vi "Load Shared Library.vi"(7 "Unload":bool, 8 "Error In":errorcluster, 11 "LabPack Shared Library In":path=path "") -> (0 "Error Out":errorcluster, 2 "Version":string, 3 "LabPack Shared Library Out":path)   [LabVIEW 2017, in "LabPack.lvlib"]
uses:
  LabPack.lvlib
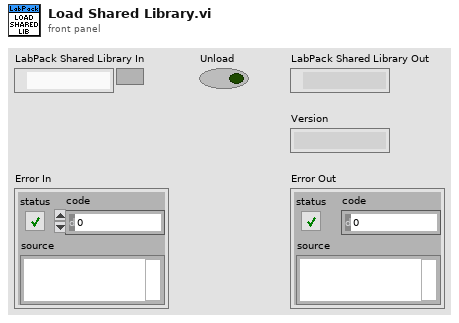
[diagram p1: front panel]
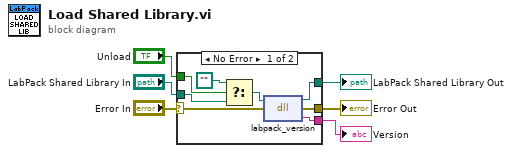
[diagram p0: block diagram]
diagram:
  n1 = case shown="No Error" "Error In" {
    selector: "Error In" -> [w7 w15]
    tunnel: "LabPack Shared Library In" -> [w13 _]
    tunnel: "Unload" -> [w11 _]
    tunnel: [w10 _] -> w4
    tunnel: [w9 _] -> w3
    tunnel: [w8 w15] -> w2
    frame No Error {
      n2 = Select(t=path "", s=w11, f=w13) -> (s? t:f=w14:path)
      n3 = dll-call lib="D:/Users/cfield/Code/MessagePack/LabPack/LabVIEW/trunk/src/LabPack/Private/labpack-x64.dll" fn="labpack_version"(path in=w14, error in=w7) -> (path out=w9:path, error out=w8:errorcluster, "return type"=w10:string)  [unwired: 1 in]
    }
    frame Error {
    }
  }
  "Version" <- w4
  "LabPack Shared Library Out" <- w3
  "Error Out" <- w2
